vi "Text_2_Optionen.vi"(8 "error in (no error)":errorcluster caption="Fehler (Eingang, kein Fehler)", 11 "Optionen String":string[][](array[string])) -> (0 "error out":errorcluster caption="Fehler (Ausgang)", 2 "Optionen":T1, 3 "Wartungsintervall:":sgl)   [LabVIEW 2020, in "System Einstellungen V2.lvlib"]
uses:
  System Einstellungen V2.lvlib
  Optionen.ctl
  <vilib>/Utility/Data Type/NI_Data Type.lvlib
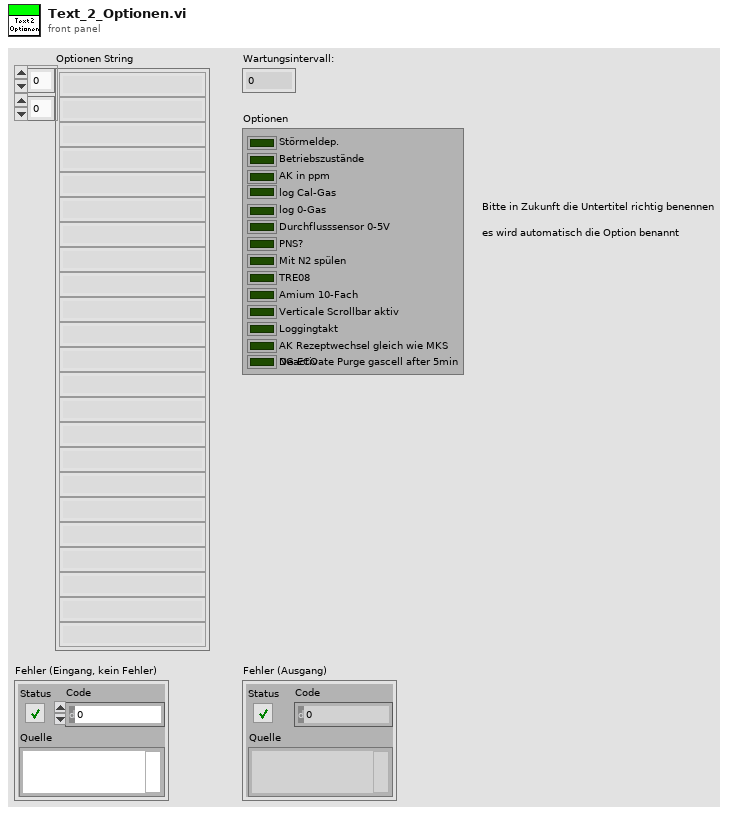
[diagram p1: front panel]
types:
  T1 = typedef "System Einstellungen V2.lvlib/Optionen.ctl" = cluster{"Störmeldep.":bool, "Betriebszustände":bool, "AK in ppm":bool, "log Cal-Gas":bool, "log 0-Gas":bool, "Durchflusssensor 0-5V":bool, "PNS?":bool, "Mit N2 spülen":bool, "TRE08":bool, "Amium 10-Fach":bool, "Verticale Scrollbar aktiv":bool, "Loggingtakt":bool, "AK Rezeptwechsel gleich wie MKS":bool, "NG ECO":bool}
  T2 = typedef "NI_Data Type.lvlib/Data Type.ctl" = enum8{"Invalid Type", "Void", "I8", "I16", "I32", "I64", "U8", "U16", "U32", "U64", "Single Float", "Double Float", "Extended Float", "Single Complex", "Double Complex", "Extended Complex", "Enum U8", "Enum U16", "Enum U32", "Enum U64", "Single Float With Unit", "Double Float With Unit", "Extended Float With Unit", "Single Complex with Unit", "Double Complex with Unit", "Extended Complex with Unit", "Boolean", "String", "Path", "Picture", "Tag", "Array", "Cluster", "Variant", "LV Variant", "Waveform", "Timestamp", "Digital Waveform", "Digital Data", "ExpressData", "Refnum", "External Data", "VI", "Poly VI", "LabVIEW Class Instance", "Fixed Point", "Set Collection", "Map Collection"}
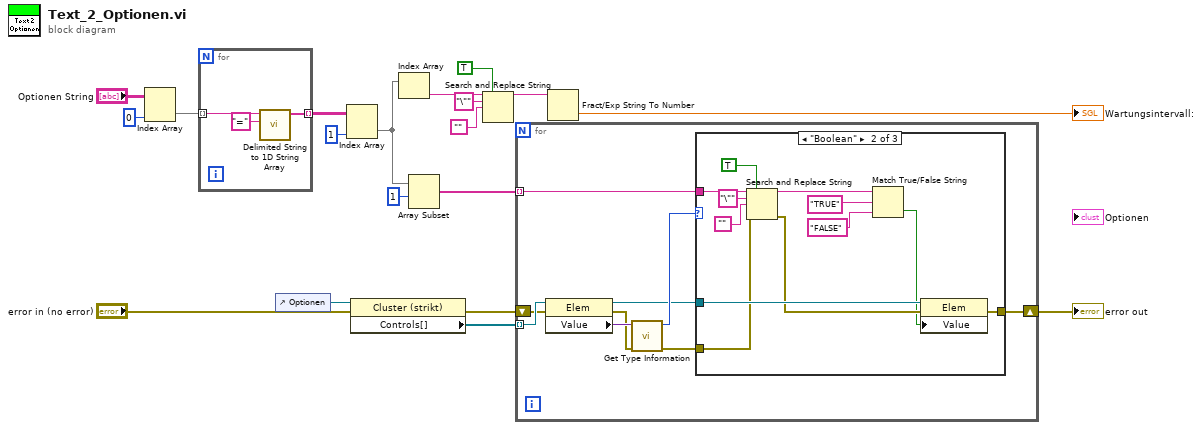
[diagram p0: block diagram]
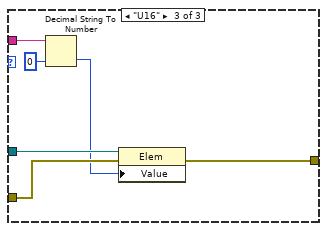
[diagram p3: hidden frame]
diagram:
  n1 = Index Array(array="Optionen String", index (col)=0 ("Deaktivierter Index (Spalte)")) -> (element=w18:string[])  [unwired: 1 in]
  n2 = for {
    tunnel: w18 -> [w22] mode=indexing
    tunnel: [w20] -> w17 mode=indexing
    n3 = call <vilib>:"Delimited String to 1D String Array.vi"("delimiter"="=", "delimited string"=w22) -> ("string array"=w20:string[])  [unwired: 9 in]
  }
  n4 = control-ref of="Optionen"() -> (w11:refnum<vi>)
  n5 = Index Array(array=w17, index (col)=1 ("Deaktivierter Index (Spalte)")) -> (element=w14:string[])  [unwired: 1 in]
  n6 = property class="Cluster (strikt)"(reference=w11, error in="error in (no error)") -> (error out=w8:errorcluster, "Controls[]"=w9:refnum<vi>[])  [unwired: 1 out]
  n7 = Index Array(array=w14) -> (element=w3:string)  [unwired: 1 in]
  n8 = Array Subset(array=w14, index=1 ("Index")) -> (w12:string[])  [unwired: 1 in]
  n9 = Search and Replace String(replace all?=TRUE ("Alle ersetzen? (F)"), input string=w3, search string="\"" ("Such-String"), replace string="") -> (result string=w1:string)  [unwired: 4 in, 3 out]
  n10 = for {
    tunnel: w12 -> [w26] mode=indexing
    tunnel: w9 -> [w31] mode=indexing
    shift-right: [w23] -> w7
    shift-left: w8 -> [w30]
    n11 = property class="Elem"(reference=w31, error in=w30) -> (reference out=w25:refnum<vi>, error out=w27:errorcluster, "Value"=w29:variant)
    n12 = call <vilib>:"Get Type Information.vi"("error in (no error)"=w27, "variant"=w29) -> ("error out"=w24:errorcluster, "type"=w28:T2)  [unwired: 5 in, 3 out]
    n13 = case shown="\"Boolean\"" w28 {
      tunnel: w26 -> [_ w42 w49]
      tunnel: w25 -> [_ w43 w48]
      tunnel: w24 -> [w32 w39 w47]
      tunnel: [w32 w44 w46] -> w23
      frame "Invalid Type", Default {
      }
      frame "Boolean" {
        n14 = Search and Replace String(replace all?=TRUE ("Alle ersetzen? (F)"), input string=w42, search string="\"" ("Such-String"), replace string="", error in=w39) -> (result string=w36:string, error out=w38:errorcluster)  [unwired: 3 in, 2 out]
        n15 = Match True/False String(2:"FALSE", 3:"TRUE", 4:w36) -> (0:w35:bool)  [unwired: 1 out]
        n16 = property class="Elem"(reference=w43, error in=w38, "Value"=w35) -> (error out=w44:errorcluster)  [unwired: 1 out]
      }
      frame "U16" {
        n17 = Decimal String To Number(string=w49, default (0L)=u16 0 ("Standard (0 I32)")) -> (number=w45:u16)  [unwired: 1 in, 1 out]
        n18 = property class="Elem"(reference=w48, error in=w47, "Value"=w45) -> (error out=w46:errorcluster)  [unwired: 1 out]
      }
    }
  }
  "error out" <- w7
  n19 = Fract/Exp String To Number(string=w1) -> (number=→"Wartungsintervall:":dbl)  [unwired: 3 in, 1 out]
